vi "Grafica.vi"() -> ()   [LabVIEW 2023]
panel:
  out "array":string[][](array[string])
  out "text":string
  out "Waveform Chart":dbl[](graph)
  out "error out 2":errorcluster
  out "error out":errorcluster
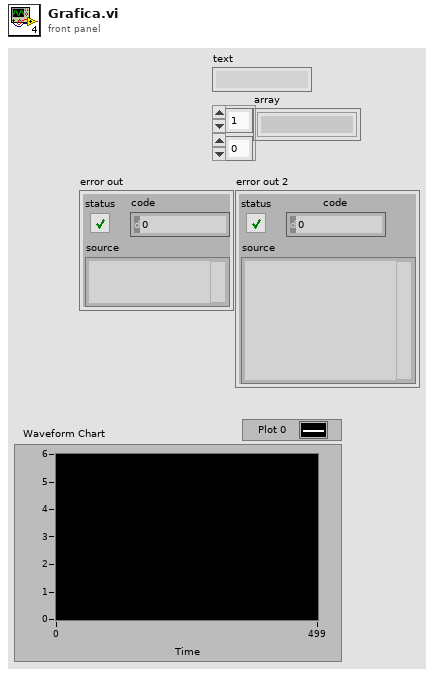
[diagram p1: front panel]
types:
  T1 = enum16{"open", "replace", "create", "open or create", "replace or create", "replace or create with confirmation"}
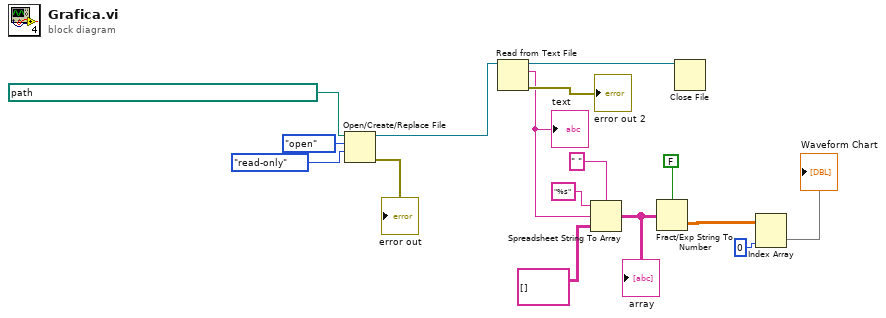
[diagram p0: block diagram]
diagram:
  n1 = Open/Create/Replace File(file path (use dialog)=path "C:/Users/chris/Downloads/señal cuadrada daq.txt", operation (0:open)=T1."open", access (0:read/write)=enum16{"read/write", "read-only", "write-only"}."read-only") -> (refnum out=w13:refnum<file>, error out=→"error out":errorcluster)  [unwired: 3 in, 1 out]
  n2 = Read from Text File(file (use dialog)=w13) -> (refnum out=w12:refnum<file>, text=w8:string, error out=→"error out 2":errorcluster)  [unwired: 3 in, 1 out]
  "text" <- w8
  n3 = Spreadsheet String To Array(delimiter (Tab)=" ", format string="%s", spreadsheet string=w8, array type (2D Dbl)=string[][] []) -> (array=w6:string[][])
  "array" <- w6
  n4 = Fract/Exp String To Number(use system decimal point (T)=FALSE, string=w6) -> (number=w3:dbl[][])  [unwired: 2 in, 1 out]
  n5 = Close File(refnum=w12) -> ()  [unwired: 1 in, 2 out]
  n6 = Index Array(array=w3, index (col)=0 ("disabled index (col)")) -> (element=→"Waveform Chart":dbl[])  [unwired: 1 in]
